vi "PH_Sound.PC PreAmp-Freigabe ein.vi"(0 "i ref in":refnum<vi>, 5 "error IO":errorcluster) -> (14 "i ref out":refnum<vi>, 19 "error out":errorcluster)   [LabVIEW 2014, in "PH_Sound.lvlib"]
doc: "This is a certain proc case."
uses:
  PH_Sound.lvlib
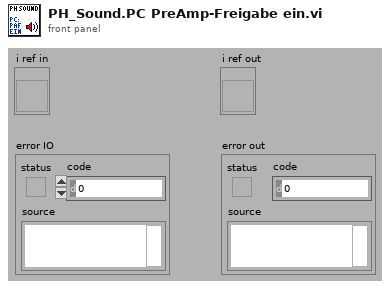
[diagram p1: front panel]
types:
  T1 = typedef "PH_Sound.lvlib/PH_Sound.i attribute.ctl" = cluster{"GUI Refs":cluster{"Exit":refnum<vi>, "Laserfreigabe":refnum<vi>, "PreAmp-Freigabe":refnum<vi>, "Countdown Running":refnum<vi>, "Emergency Off":refnum<vi>, "Device Error":refnum<vi>}, "Testalarm on":bool, "State":cluster{"Laser Class 4":bool, "PreAmp Running":bool, "Countdown Running":bool, "Emergency Off":bool}, "Starting Time":timestamp}
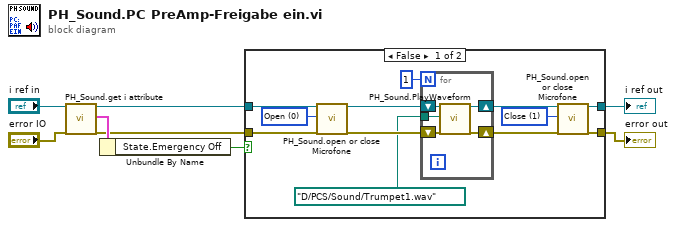
[diagram p0: block diagram]
diagram:
  n1 = call "PH_Sound.get i attribute.vi"("i ref in"="i ref in", "error in (no error)"="error IO") -> ("i ref out"=w2:refnum<vi>, "i attribute"=w3:T1, "error out"=w1:errorcluster)  [unwired: 15 in]
  n2 = Unbundle By Name(w3) -> ("State.Emergency Off"=w6:bool)
  n3 = case shown="False" w6 {
    tunnel: [w16 w27] -> w8
    tunnel: [w17 w26] -> w7
    tunnel: w1 -> [w19 w26]
    tunnel: w2 -> [w20 w27]
    frame False {
      w15 = u16 1 items=["Open", "Close"] ("Action")
      w18 = u16 0 items=["Open", "Close"] ("Action")
      n4 = call "PH_Sound.open or close Microfone.vi"("i ref in"=w20, "Action"=w18, "error in (no error)"=w19) -> ("i ref out"=w10:refnum<vi>, "error out"=w11:errorcluster)  [unwired: 15 in]
      n5 = for {
        N: 1 -> [_]
        tunnel: path "D:/PCS/Sound/Trumpet1.wav" ("path") -> [w21]
        shift-right: [w22] -> w12
        shift-left: w10 -> [w23]
        shift-right: [w24] -> w13
        shift-left: w11 -> [w25]
        n6 = call "PH_Sound.PlayWaveform.vi"("i ref in"=w23, "path"=w21, "error in (no error)"=w25) -> ("i ref out"=w22:refnum<vi>, "error out"=w24:errorcluster)  [unwired: 15 in]
      }
      n7 = call "PH_Sound.open or close Microfone.vi"("i ref in"=w12, "Action"=w15, "error in (no error)"=w13) -> ("i ref out"=w16:refnum<vi>, "error out"=w17:errorcluster)  [unwired: 15 in]
    }
    frame True {
    }
  }
  "i ref out" <- w8
  "error out" <- w7
